vi "main.vi"() -> ()   [LabVIEW 2014]
uses:
  <vilib>/Instr/_visa.llb/VISA Configure Serial Port (Instr).vi
  <instrlib>/Keithley 24XX/Public/Data/Read (Multiple Points).vi
  <instrlib>/Keithley 24XX/Keithley 24XX.lvlib
panel:
  out "Data IV Keithley":string
  in  "Data IV Keithley 2":path=path "C:/Users/Administrator/Documents/Device-characterization-setup/IV-Trace/Data/dumb/2015_xx_xx_xxxx_xx_keithley_001.txt"
  out "IV Curve":cluster{"Voltage":sgl[], "Current":sgl[]}(graph)
  out "Data Resistivity":string
  in  "Data Resistivity  2":path=path "C:/Users/Administrator/Documents/Device-characterization-setup/IV-Trace/Data/dumb/2015_xx_xx_xxxx_xx_keithley_resistivity_001.txt"
  out "Resistance-Voltage":cluster{sgl[], sgl[]}(graph)
  in  "Source Mode  (0: Voltage)":u16(ring) items=["Voltage", "Current"]
  in  "Serial Configuration":T1={"Baud Rate"=9600, "Parity"=0, "Data Bits"=8, "Stop Bits"=10, "Flow Control"=0} {"Flow Control" items=["None", "XON/XOFF", "RTS/CTS", "XON/XOFF & RTS/CTS", "DTR/DSR", "XON/XOFF & DTR/DSR"]; "Stop Bits" items=["1.0"=10, "1.5"=15, "2.0"=20]; "Data Bits" items=["7"=7, "8"=8]; "Parity" items=["None", "Odd", "Even", "Mark", "Space"]; "Baud Rate" items=["300"=300, "600"=600, "1200"=1200, "2400"=2400, "4800"=4800, "9600"=9600, "19200"=19200]}
  in  "VISA resource name":refnum<visa-resource-name>="GPIB9::24::INSTR"
  in  "Timeout (10000 ms)":i32=10000 format="%#.6g"
  in  "Maximum Amplitude (2)":dbl=2.0
  in  "Minimum Amplitude (1)":dbl=1.0
  in  "Number of Points (5)":u32=5
  in  "Compliance  Level (1)":dbl=1.0
  out "Seconds":sgl
  out "Chamber *C Data":string
  in  "Chamber *C Data":path=path "C:/Users/Administrator/Documents/humidity_sensing_setup/data/dumb/chamber_c_data.txt"
  out "Chamber *C Graph":sgl(graph)=5460.51
  out "Chamber *C":sgl
  out "Thermocouple Temperature Graph":sgl(graph)=5460.51
  out "Thermocouple Temperature":sgl
  out "Thermocouple *C Data":string
  in  "Thermocouple *C Data":path=path "C:/Users/Administrator/Documents/humidity_sensing_setup/data/dumb/thermocouple_c_data.txt"
  out "Pressure Data":string
  in  "Pressure Data":path=path "C:/Users/Administrator/Documents/humidity_sensing_setup/data/dumb/pressure_data.txt"
  out "Pressure Graph":sgl(graph)=5460.51
  out "Pressure":sgl
  in  "Start Button":bool
  out "Humidity":sgl
  out "Humidity Data":string
  in  "Humidity Data":path=path "C:/Users/Administrator/Documents/humidity_sensing_setup/data/dumb/humidity_data.txt"
  out "Humidity Data Graph":sgl(graph)=5460.51
  in  "Sampling rate (ms/pt)":i32=1000
  in  "stop button":bool
  in  "loop num":dbl=10000000000.0
  out "Arduino Status":bool
  out "error out":errorcluster
  in  "error in":errorcluster
  in  "instr name":string="Arduino"
  in  "write":bool
  in  "buffer size":u32=256
  in  "timeout (ms)":u32=10000
  in  "flow control":u16
  in  "stop bits":u16=10
  in  "parity":u16(ring) items=["None", "Odd", "Even", "Mark", "Space"]
  in  "data bits":u16=8 min=5 max=8 step=1
  in  "baud rate":u32=9600
  in  "write string":string
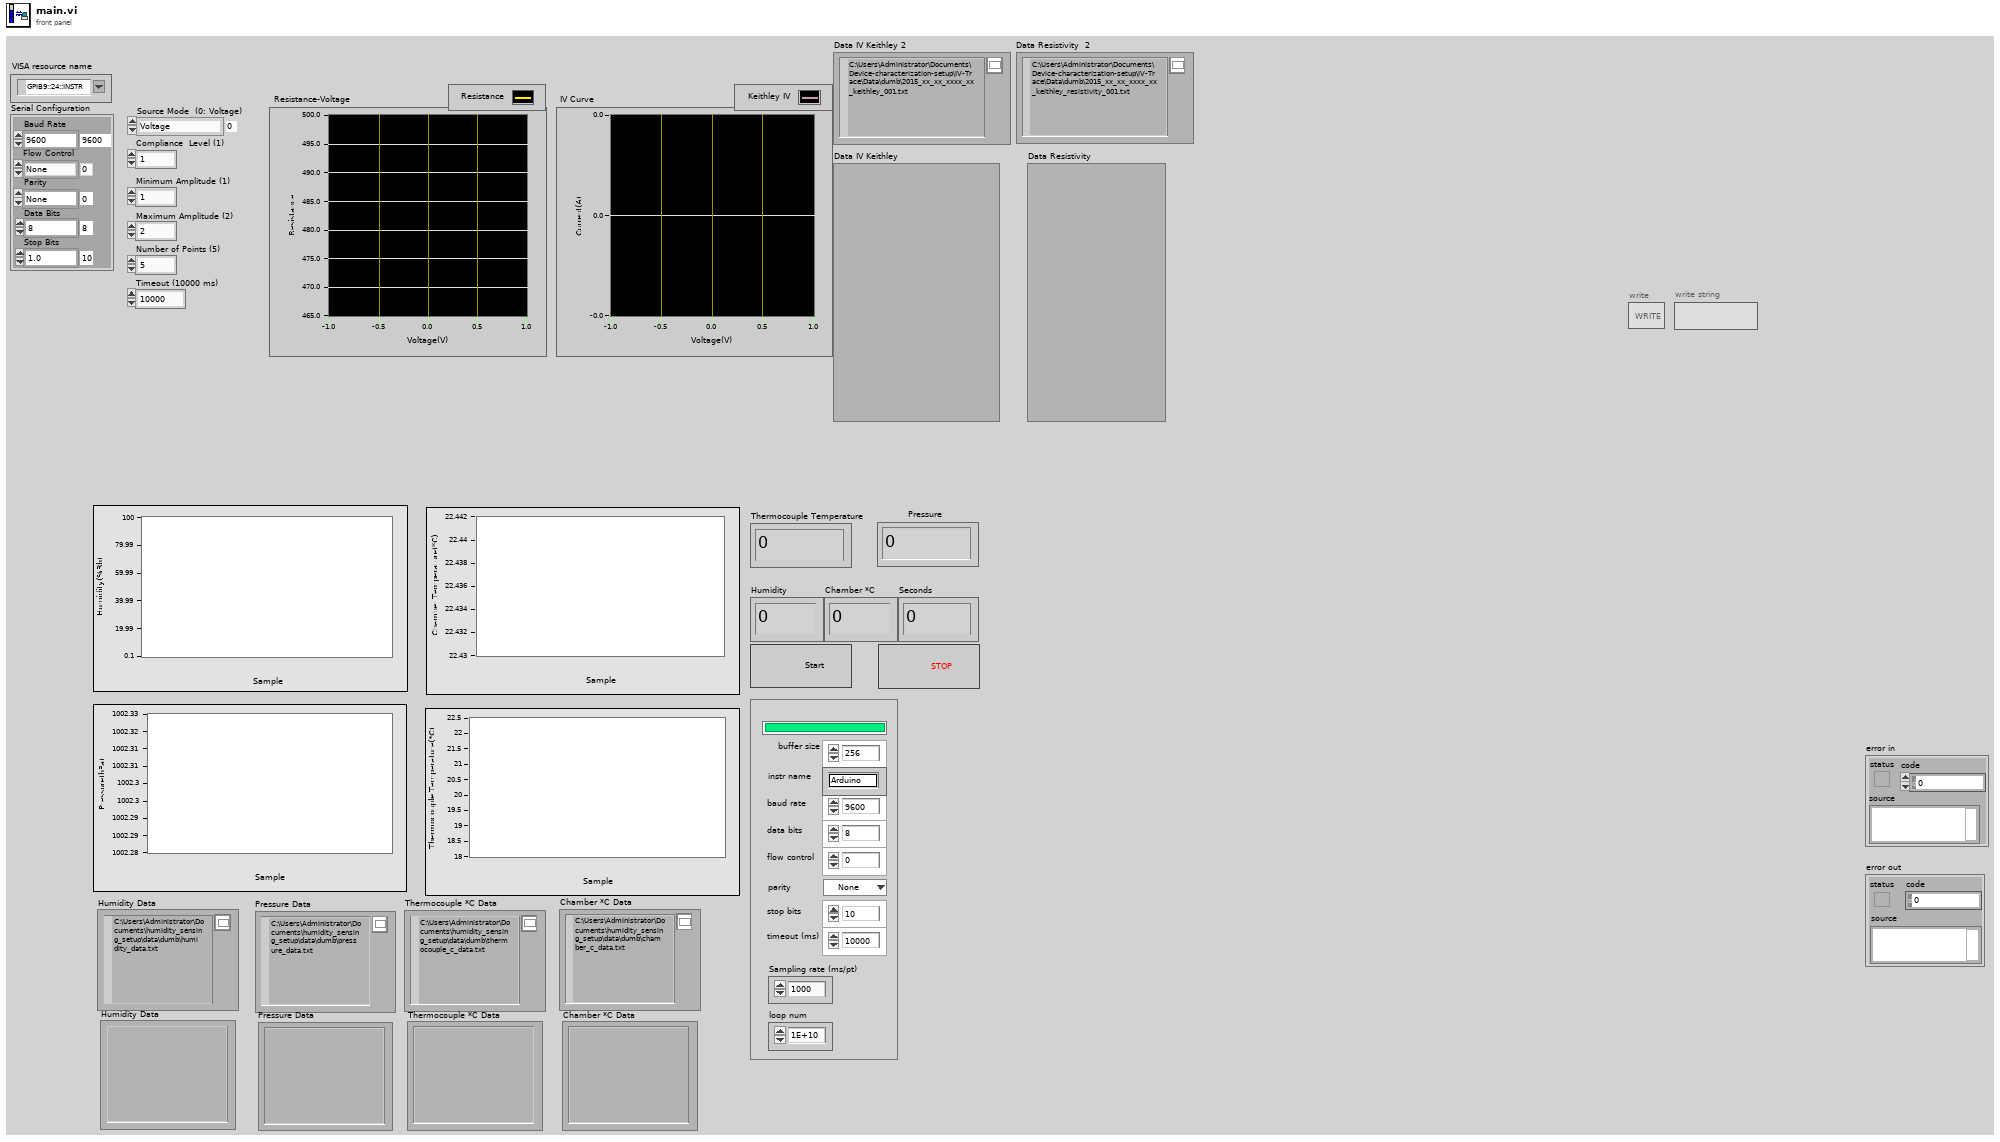
[diagram p1: front panel]
types:
  T1 = cluster{"Baud Rate":u32, "Parity":u16, "Data Bits":u16, "Stop Bits":u16, "Flow Control":u16}
  T2 = enum16{"open", "replace", "create", "open or create", "replace or create", "replace or create with confirmation"}
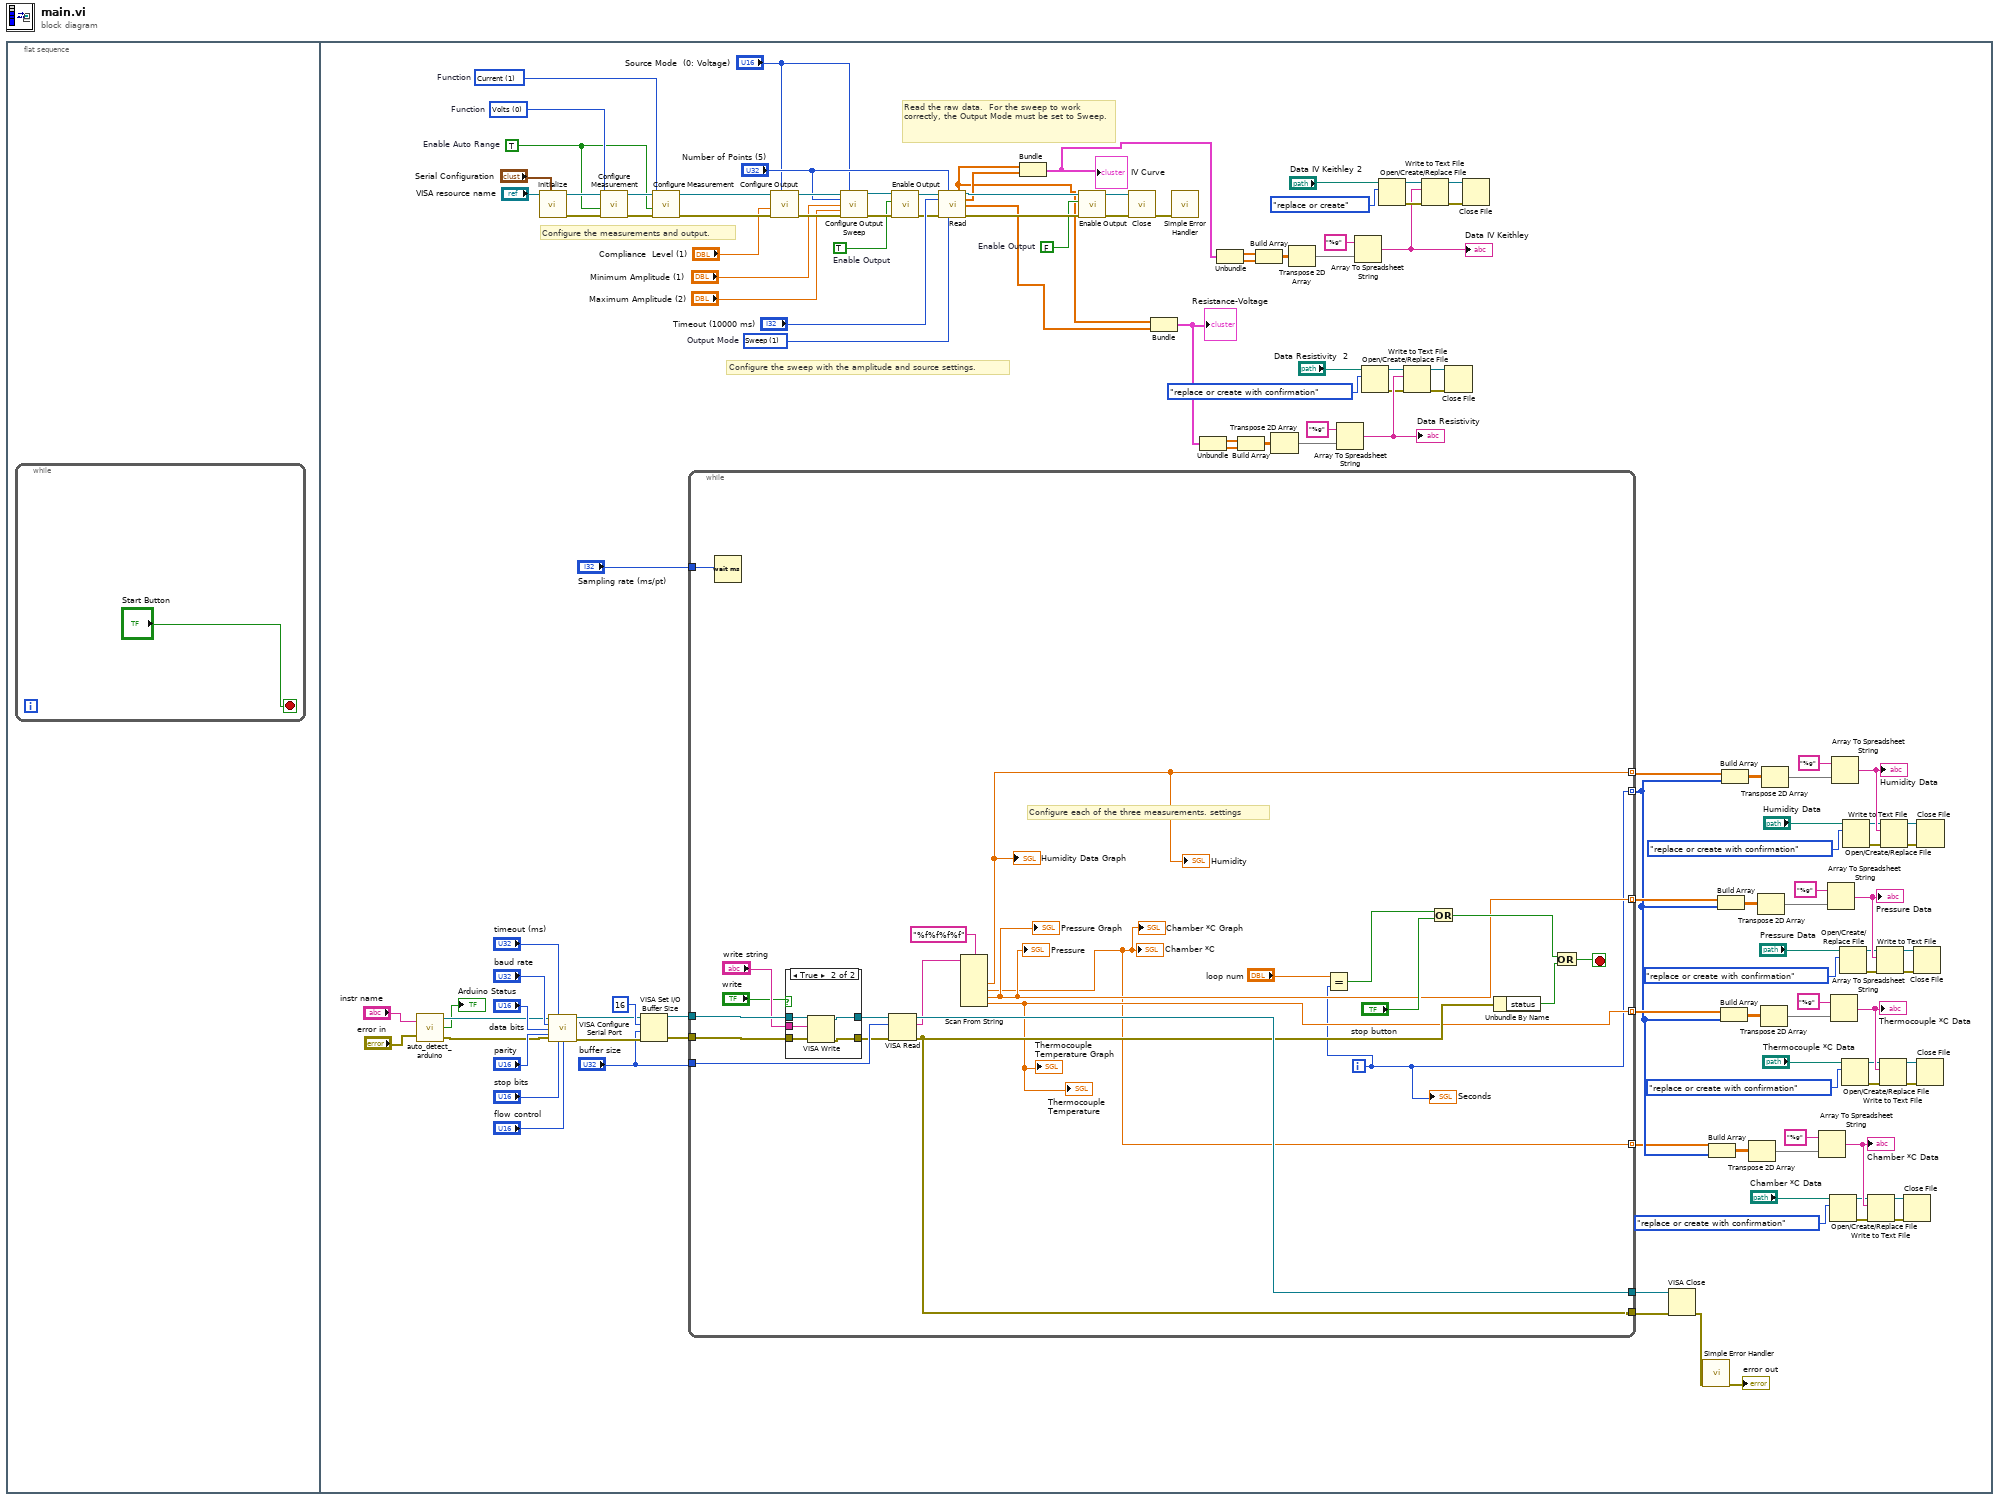
[diagram p0: block diagram]
diagram:
  n1 = flat-sequence {
    frame #0 {
      n2 = while {
        stop <- "Start Button" stop-if-true
      }
    }
    frame #1 {
      w32 = TRUE  # Enable Output
      w33 = TRUE  # Enable Auto Range
      w34 = u16 1 items=["Volts", "Current", "Resistance"]  # Function
      w35 = u16 0 items=["Volts", "Current", "Resistance"]  # Function
      w41 = FALSE  # Enable Output
      w47 = u16 1 items=["Fixed", "Sweep", "List"]  # Output Mode
      # "Read the raw data.  For the sweep to work correctly, the Output Mode must be set to Sweep."
      # "Configure the sweep with the amplitude and source settings."
      # "Configure the measurements and output."
      n3 = call "auto_detect_arduino.vi"("instr name"="instr name", "error in"="error in") -> ("VISA resource name"=w120:refnum<visa-resource-name>, "status"=→"Arduino Status":bool, "error out"=w119:errorcluster)
      n4 = call <instrlib>:"Initialize.vi"("Serial Configuration"="Serial Configuration", "VISA resource name"="VISA resource name") -> ("error out"=w60:errorcluster, "VISA resource name out"=w61:refnum<visa-resource-name>)  [unwired: 8 in]
      n5 = call-poly "VISA Configure Serial Port"("VISA resource name"=w120, "timeout (10sec)"="timeout (ms)", "baud rate (9600)"="baud rate", "data bits (8)"="data bits", "parity (0:none)"="parity", "error in (no error)"=w119, "stop bits (10: 1 bit)"="stop bits", "flow control (0:none)"="flow control") -> ("VISA resource name out"=w116:refnum<visa-resource-name>, "error out"=w115:errorcluster)  [unwired: 6 in]
      n6 = call <instrlib>:"Configure Measurement.vi"("error in (no error)"=w60, "Enable Auto Range (T:Enable)"=w33, "Function (0: Volts)"=w35, "VISA resource name"=w61) -> ("error out"=w59:errorcluster, "VISA resource name out"=w58:refnum<visa-resource-name>)  [unwired: 6 in]
      n7 = VISA Set I/O Buffer Size(VISA resource name=w116, mask (16)=u16 16 ("I/O Receive\nBuffer mask"), size (4096)="buffer size", error in (no error)=w115) -> (VISA resource name out=w114:refnum<visa-resource-name>, error out=w113:errorcluster)
      n8 = call <instrlib>:"Configure Measurement.vi"("error in (no error)"=w59, "Enable Auto Range (T:Enable)"=w33, "Function (0: Volts)"=w34, "VISA resource name"=w58) -> ("error out"=w56:errorcluster, "VISA resource name out"=w57:refnum<visa-resource-name>)  [unwired: 6 in]
      n9 = while {
        tunnel: w114 -> [w148]
        tunnel: w113 -> [w147]
        tunnel: [w149] -> w128
        tunnel: [w137] -> w127
        tunnel: "buffer size" -> [w150]
        tunnel: [w138] -> w96 mode=indexing
        tunnel: "Sampling rate (ms/pt)" -> [w140]
        tunnel: [w130] -> w63 mode=indexing
        tunnel: [w133] -> w85 mode=indexing
        tunnel: [w132] -> w74 mode=indexing
        tunnel: [w131] -> w62 mode=indexing
        i -> [w130]
        stop <- w151 stop-if-true
        # "Configure each of the three measurements. settings"
        n10 = Wait (ms)(milliseconds to wait=w140) -> ()  [unwired: 1 out]
        n11 = case shown="True" "write" {
          tunnel: w148 -> [w153 w158]
          tunnel: w147 -> [w152 w157]
          tunnel: [w153 w156] -> w146
          tunnel: [w152 w155] -> w145
          tunnel: "write string" -> [_ w154]
          frame False {
          }
          frame True {
            n12 = VISA Write(VISA resource name=w158, write buffer=w154, error in (no error)=w157) -> (VISA resource name out=w156:refnum<visa-resource-name>, error out=w155:errorcluster)  [unwired: 1 out]
          }
        }
        n13 = VISA Read(VISA resource name=w146, byte count=w150, error in (no error)=w145) -> (VISA resource name out=w149:refnum<visa-resource-name>, read buffer=w134:string, error out=w137:errorcluster)  [unwired: 1 out]
        n14 = Scan From String(format string="%f%f%f%f", input string=w134) -> (output 1=w138:sgl, output 2=w131:sgl, output 3=w133:sgl, output 4=w132:sgl)  [unwired: 6 in, 3 out]
        "Humidity Data Graph" <- w138
        "Humidity" <- w138
        "Pressure" <- w133
        "Pressure Graph" <- w133
        "Thermocouple Temperature" <- w132
        "Thermocouple Temperature Graph" <- w132
        "Chamber *C" <- w131
        "Chamber *C Graph" <- w131
        n15 = Equal?(x="loop num", y=w130) -> (x = y?=w129:bool)
        n16 = Or(x=w129, y="stop button") -> (x .or. y?=w135:bool)
        n17 = Unbundle By Name(w137) -> ("status"=w136:bool)
        n18 = Or(x=w135, y=w136) -> (x .or. y?=w151:bool)
        "Seconds" <- w130
      }
      n19 = call <instrlib>:"Configure Output.vi"("Source Mode  (0: Voltage)"="Source Mode  (0: Voltage)", "error in (no error)"=w56, "Compliance  Level (0.1)"="Compliance  Level (1)", "VISA resource name"=w57) -> ("error out"=w55:errorcluster, "VISA resource name out"=w54:refnum<visa-resource-name>)  [unwired: 6 in]
      n20 = call <instrlib>:"Configure Output Sweep.vi"("VISA resource name"=w54, "Source Mode  (0: Voltage)"="Source Mode  (0: Voltage)", "Number of Points (5)"="Number of Points (5)", "Minimum Amplitude (1)"="Minimum Amplitude (1)", "Maximum Amplitude (2)"="Maximum Amplitude (2)", "error in (no error)"=w55) -> ("VISA resource name out"=w38:refnum<visa-resource-name>, "error out"=w37:errorcluster)  [unwired: 8 in]
      n21 = call <instrlib>:"Enable Output.vi"("error in (no error)"=w37, "Enable Output (T: Enable)"=w32, "VISA resource name"=w38) -> ("error out"=w40:errorcluster, "VISA resource name out"=w39:refnum<visa-resource-name>)  [unwired: 7 in]
      n22 = call-poly <instrlib>:"Read.vi"("VISA resource name"=w39, "Sample Count (1)"="Number of Points (5)", "Timeout (10000 ms)"="Timeout (10000 ms)", "error in (no error)"=w40, "Output Mode (0: Fixed)"=w47) -> ("Voltage"=w5:sgl[], "VISA resource name out"=w42:refnum<visa-resource-name>, "Current"=w30:sgl[], "Resistance"=w6:sgl[], "error out"=w43:errorcluster)  [unwired: 4 in, 2 out]
      n23 = Bundle("Voltage"=w5, "Current"=w30) -> (w4:cluster{"Voltage":sgl[], "Current":sgl[]})  [unwired: 1 out]
      "IV Curve" <- w4
      n24 = call <instrlib>:"Enable Output.vi"("error in (no error)"=w43, "Enable Output (T: Enable)"=w41, "VISA resource name"=w42) -> ("error out"=w44:errorcluster, "VISA resource name out"=w45:refnum<visa-resource-name>)  [unwired: 7 in]
      n25 = call <instrlib>:"Close.vi"("error in (no error)"=w44, "VISA resource name"=w45) -> ("error out"=w46:errorcluster)  [unwired: 9 in]
      n26 = Bundle("Voltage"=w5, "Resistance"=w6) -> (w13:cluster{"Voltage":sgl[], "Resistance":sgl[]})  [unwired: 1 out]
      "Resistance-Voltage" <- w13
      n27 = call <vilib>:"Simple Error Handler.vi"("error in (no error)"=w46) -> ()  [unwired: 4 in, 5 out]
      n28 = Unbundle(w13) -> ("Voltage"=w14:sgl[], "Resistance"=w15:sgl[])
      n29 = Unbundle(w4) -> ("Voltage"=w25:sgl[], "Current"=w26:sgl[])
      n30 = Build Array(w14, w15) -> (w16:sgl[][])
      n31 = Build Array(w25, w26) -> (w27:sgl[][])
      n32 = Transpose 2D Array(2D array=w16) -> (transposed array=w18:sgl[][])
      n33 = Transpose 2D Array(2D array=w27) -> (transposed array=w29:sgl[][])
      n34 = Array To Spreadsheet String(array=w18, 3:"%g" ("format string")) -> (spreadsheet string=w19:string)  [unwired: 1 in]
      "Data Resistivity" <- w19
      n35 = Array To Spreadsheet String(array=w29, 3:"%g" ("format string")) -> (spreadsheet string=w2:string)  [unwired: 1 in]
      "Data IV Keithley" <- w2
      n36 = Open/Create/Replace File(file path (use dialog)="Data Resistivity  2", operation (0:open)=T2."replace or create with confirmation") -> (refnum out=w12:refnum<file>, error out=w7:errorcluster)  [unwired: 4 in, 1 out]
      n37 = Open/Create/Replace File(file path (use dialog)="Data IV Keithley 2", operation (0:open)=T2."replace or create") -> (refnum out=w24:refnum<file>, error out=w20:errorcluster)  [unwired: 4 in, 1 out]
      n38 = Write to Text File(file (use dialog)=w12, text=w19, error in=w7) -> (refnum out=w9:refnum<file>, error out=w8:errorcluster)  [unwired: 2 out]
      n39 = Write to Text File(file (use dialog)=w24, text=w2, error in=w20) -> (refnum out=w22:refnum<file>, error out=w21:errorcluster)  [unwired: 2 out]
      n40 = Close File(refnum=w9, error in=w8) -> ()  [unwired: 2 out]
      n41 = Close File(refnum=w22, error in=w21) -> ()  [unwired: 2 out]
      n42 = VISA Close(VISA resource name=w128, error in (no error)=w127) -> (error out=w110:errorcluster)
      n43 = call <vilib>:"Simple Error Handler.vi"("error in (no error)"=w110) -> ("error out"=→"error out":errorcluster)  [unwired: 4 in, 4 out]
      n44 = Build Array(w62, w63) -> (w64:sgl[][])
      n45 = Build Array(w85, w63) -> (w86:sgl[][])
      n46 = Build Array(w74, w63) -> (w75:sgl[][])
      n47 = Build Array(w96, w63) -> (w97:sgl[][])
      n48 = Transpose 2D Array(2D array=w64) -> (transposed array=w72:sgl[][])
      n49 = Transpose 2D Array(2D array=w86) -> (transposed array=w94:sgl[][])
      n50 = Transpose 2D Array(2D array=w75) -> (transposed array=w83:sgl[][])
      n51 = Transpose 2D Array(2D array=w97) -> (transposed array=w105:sgl[][])
      n52 = Array To Spreadsheet String(array=w72, 3:"%g" ("format string")) -> (spreadsheet string=w73:string)  [unwired: 1 in]
      "Chamber *C Data" <- w73
      n53 = Array To Spreadsheet String(array=w94, 3:"%g" ("format string")) -> (spreadsheet string=w95:string)  [unwired: 1 in]
      "Pressure Data" <- w95
      n54 = Open/Create/Replace File(file path (use dialog)="Chamber *C Data", operation (0:open)=T2."replace or create with confirmation") -> (refnum out=w70:refnum<file>, error out=w65:errorcluster)  [unwired: 4 in, 1 out]
      n55 = Array To Spreadsheet String(array=w83, 3:"%g" ("format string")) -> (spreadsheet string=w84:string)  [unwired: 1 in]
      "Thermocouple *C Data" <- w84
      n56 = Array To Spreadsheet String(array=w105, 3:"%g" ("format string")) -> (spreadsheet string=w106:string)  [unwired: 1 in]
      "Humidity Data" <- w106
      n57 = Open/Create/Replace File(file path (use dialog)="Pressure Data", operation (0:open)=T2."replace or create with confirmation") -> (refnum out=w92:refnum<file>, error out=w87:errorcluster)  [unwired: 4 in, 1 out]
      n58 = Open/Create/Replace File(file path (use dialog)="Thermocouple *C Data", operation (0:open)=T2."replace or create with confirmation") -> (refnum out=w81:refnum<file>, error out=w76:errorcluster)  [unwired: 4 in, 1 out]
      n59 = Open/Create/Replace File(file path (use dialog)="Humidity Data", operation (0:open)=T2."replace or create with confirmation") -> (refnum out=w103:refnum<file>, error out=w98:errorcluster)  [unwired: 4 in, 1 out]
      n60 = Write to Text File(file (use dialog)=w70, text=w73, error in=w65) -> (refnum out=w67:refnum<file>, error out=w66:errorcluster)  [unwired: 2 out]
      n61 = Write to Text File(file (use dialog)=w92, text=w95, error in=w87) -> (refnum out=w89:refnum<file>, error out=w88:errorcluster)  [unwired: 2 out]
      n62 = Write to Text File(file (use dialog)=w81, text=w84, error in=w76) -> (refnum out=w78:refnum<file>, error out=w77:errorcluster)  [unwired: 2 out]
      n63 = Write to Text File(file (use dialog)=w103, text=w106, error in=w98) -> (refnum out=w100:refnum<file>, error out=w99:errorcluster)  [unwired: 2 out]
      n64 = Close File(refnum=w67, error in=w66) -> ()  [unwired: 2 out]
      n65 = Close File(refnum=w89, error in=w88) -> ()  [unwired: 2 out]
      n66 = Close File(refnum=w78, error in=w77) -> ()  [unwired: 2 out]
      n67 = Close File(refnum=w100, error in=w99) -> ()  [unwired: 2 out]
    }
  }
